vi "write header.vi"(8 "error in (no error)":errorcluster, 10 "line #":i32, 11 "Byte Stream File in":refnum<file>) -> (0 "error out":errorcluster, 3 "Byte Stream File out":refnum<file>)   [LabVIEW 2014, in "PLS Logging.lvlib"]
uses:
  PLS Logging.lvlib
  support/GLB_PAmonts.vi
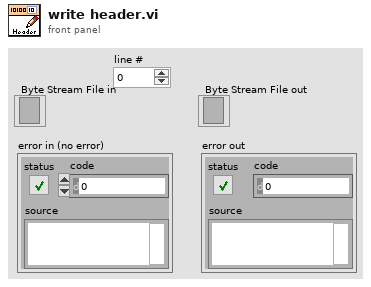
[diagram p1: front panel]
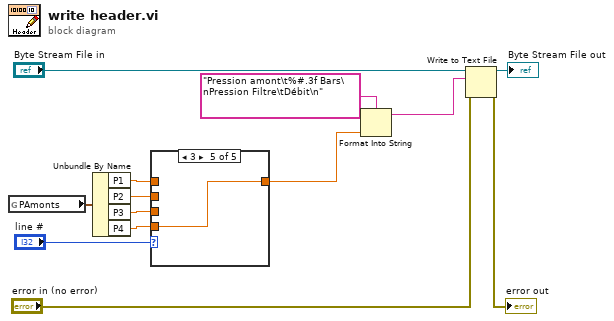
[diagram p0: block diagram]
diagram:
  n1 = global read "GLB_PAmonts.vi" "PAmonts"() -> (w9:cluster{"P1":dbl, "P2":dbl, "P3":dbl, "P4":dbl})
  n2 = Unbundle By Name(w9) -> ("P1"=w7:dbl, "P2"=w6:dbl, "P3"=w5:dbl, "P4"=w4:dbl)
  n3 = case shown="3" "line #" {
    tunnel: w7 -> [w14 w15 _ _ _]
    tunnel: w6 -> [_ _ w16 _ _]
    tunnel: w5 -> [_ _ _ w17 _]
    tunnel: w4 -> [_ _ _ _ w18]
    tunnel: [w14 w15 w16 w17 w18] -> w3
    frame Default {
    }
    frame 0 {
    }
    frame 1 {
    }
    frame 2 {
    }
    frame 3 {
    }
  }
  n4 = Format Into String(format string="Pression amont\t%#.3f Bars\nPression Filtre\tDébit\n", w3) -> (resulting string=w2:string)  [unwired: 2 in, 1 out]
  n5 = Write to Text File(file (use dialog)="Byte Stream File in", text=w2, error in="error in (no error)") -> (refnum out=→"Byte Stream File out":refnum<file>, error out=→"error out":errorcluster)  [unwired: 1 in, 1 out]
